vi "CONFIG FILE MAIN Unitest.vi"(0 "File Path":path, 1 "WRITE /READ SECTION":string, 2 "READ KEY":string, 3 "WRITE KEY":string, 4 "WRITE VALUE":string, 5 "error in":errorcluster, 6 "file name":string=".ini", 7 "PARAMETER/CONFIG":bool, 8 "Config Enum":T1) -> (15 "READ VALUE":string, 19 "error out":errorcluster)   [LabVIEW 2025]
uses:
  Config file  FGV Unitest enum.ctl
  <vilib>/Utility/config.llb/Read Key (String).vi
  <vilib>/Utility/config.llb/Write Key (String).vi
  <vilib>/Utility/config.llb/NI_LVConfig.lvlib
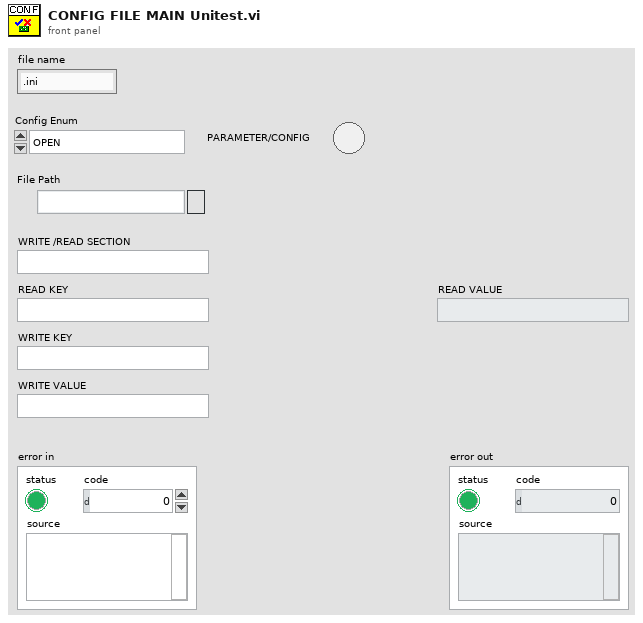
[diagram p1: front panel]
types:
  T1 = typedef "Config file  FGV Unitest enum.ctl" = enum16{"OPEN", "READ", "WRITE", "CLOSE"}
  T2 = typedef "NI_LVConfig.lvlib/Config Data RefNum.ctl" = refnum<k1>
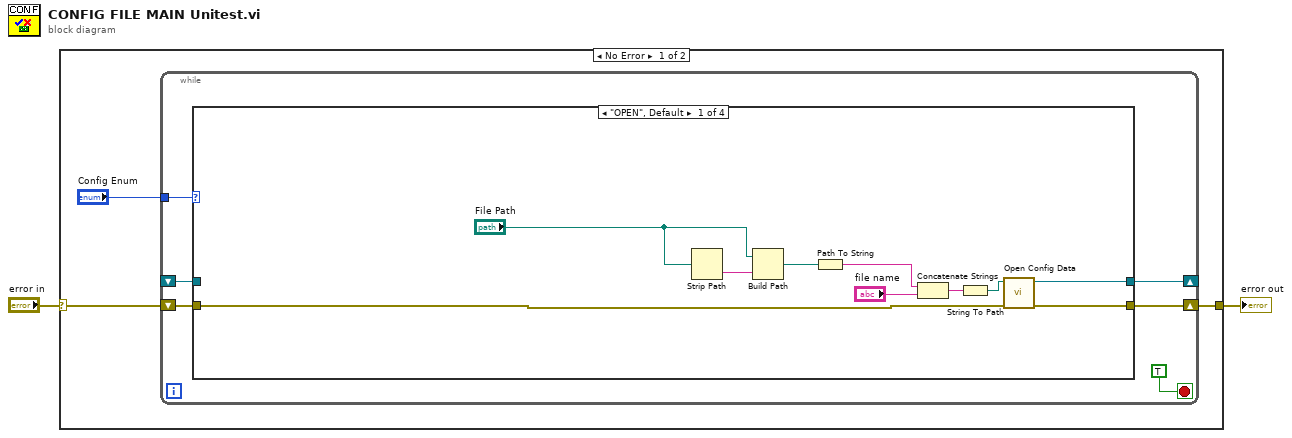
[diagram p0: block diagram]
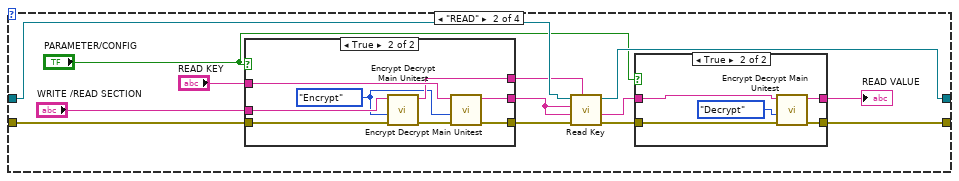
[diagram p2: hidden frame]
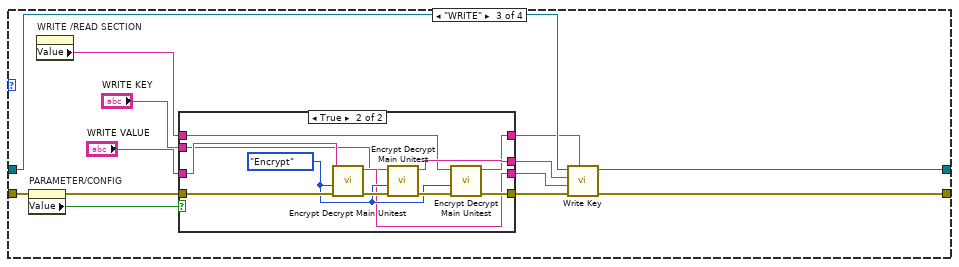
[diagram p5: hidden frame]
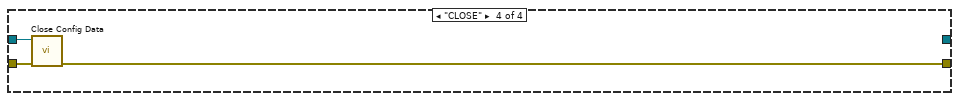
[diagram p7: hidden frame]
diagram:
  n1 = case shown="No Error" "error in" {
    selector: "error in" -> [w4 _]
    tunnel: [w3 _] -> w1
    frame No Error {
      n2 = while {
        tunnel: "Config Enum" -> [w11]
        shift-right: [w9] -> w3
        shift-left: w4 -> [w10]
        shift-right: [w8] -> _
        shift-left: _ -> [w6]
        stop <- TRUE stop-if-true
        n3 = case shown="\"OPEN\", Default" w11 {
          tunnel: w10 -> [w21 w32 w55 w83]
          tunnel: [w20 w25 w64 w81] -> w9
          tunnel: [w19 w33 w63 _] -> w8
          tunnel: w6 -> [_ w34 w65 w82]
          frame "OPEN", Default {
            n4 = Strip Path(path="File Path") -> (name=w13:string)  [unwired: 1 out]
            n5 = Build Path(base path="File Path", name or relative path=w13) -> (appended path=w12:path)
            n6 = Path To String(path=w12) -> (string=w18:string)
            n7 = Concatenate Strings(w18, "file name") -> (w16:string)
            n8 = String To Path(string=w16) -> (path=w15:path)
            n9 = call <vilib>:"Open Config Data.vi"("error in (no error)"=w21, "configuration file path"=w15) -> ("error out"=w20:errorcluster, "refnum"=w19:T2)  [unwired: 7 in, 1 out]
          }
          frame "READ" {
            n10 = case shown="True" "PARAMETER/CONFIG" {
              tunnel: w32 -> [w35 w45]
              tunnel: [w35 w43] -> w31
              tunnel: [w36 w42] -> w30
              tunnel: "READ KEY" -> [w36 w41]
              tunnel: [w37 w40] -> w28
              tunnel: "WRITE /READ SECTION" -> [w37 w39]
              frame False {
              }
              frame True {
                w38 = enum16{"Decrypt", "Encrypt"}."Encrypt" ("Process")
                n11 = call "Encrypt Decrypt Main Unitest.vi"("error in (no error)"=w45, "Process"=w38, "Input"=w39) -> ("error out"=w44:errorcluster, "Output"=w40:string)  [unwired: 7 in]
                n12 = call "Encrypt Decrypt Main Unitest.vi"("error in (no error)"=w44, "Process"=w38, "Input"=w41) -> ("error out"=w43:errorcluster, "Output"=w42:string)  [unwired: 7 in]
              }
            }
            n13 = call-poly <vilib>:"Read Key.vi"("section"=w28, "error in (no error)"=w31, "default value"=w30, "key"=w30, "refnum"=w34) -> ("error out"=w26:errorcluster, "value"=w24:string, "refnum out"=w33:T2)  [unwired: 3 in, 1 out]
            n14 = case shown="True" "PARAMETER/CONFIG" {
              tunnel: w26 -> [w47 w52]
              tunnel: [w47 w51] -> w25
              tunnel: w24 -> [w46 w50]
              tunnel: [w46 w49] -> w23
              frame False {
              }
              frame True {
                n15 = call "Encrypt Decrypt Main Unitest.vi"("error in (no error)"=w52, "Process"=enum16{"Decrypt", "Encrypt"}."Decrypt", "Input"=w50) -> ("error out"=w51:errorcluster, "Output"=w49:string)  [unwired: 7 in]
              }
            }
            "READ VALUE" <- w23
          }
          frame "WRITE" {
            n16 = property on="PARAMETER/CONFIG" class="Bool (strict)"(error in=w55) -> (error out=w54:errorcluster, "Value"=w53:bool)  [unwired: 1 in, 1 out]
            n17 = property on="WRITE /READ SECTION" class="Str"() -> ("Value"=w57:string)  [unwired: 2 in, 2 out]
            n18 = case shown="True" w53 {
              tunnel: w54 -> [w66 w80]
              tunnel: [w66 w77] -> w62
              tunnel: [w67 w75] -> w61
              tunnel: "WRITE VALUE" -> [w67 w74]
              tunnel: [w68 w73] -> w59
              tunnel: "WRITE KEY" -> [w68 w72]
              tunnel: w57 -> [w69 w71]
              tunnel: [w69 w70] -> w56
              frame False {
              }
              frame True {
                w76 = enum16{"Decrypt", "Encrypt"}."Encrypt" ("Process")
                n19 = call "Encrypt Decrypt Main Unitest.vi"("error in (no error)"=w80, "Process"=w76, "Input"=w74) -> ("error out"=w79:errorcluster, "Output"=w75:string)  [unwired: 7 in]
                n20 = call "Encrypt Decrypt Main Unitest.vi"("error in (no error)"=w79, "Process"=w76, "Input"=w72) -> ("error out"=w78:errorcluster, "Output"=w73:string)  [unwired: 7 in]
                n21 = call "Encrypt Decrypt Main Unitest.vi"("error in (no error)"=w78, "Process"=w76, "Input"=w71) -> ("error out"=w77:errorcluster, "Output"=w70:string)  [unwired: 7 in]
              }
            }
            n22 = call-poly <vilib>:"Write Key.vi"("section"=w56, "error in (no error)"=w62, "value"=w61, "key"=w59, "refnum"=w65) -> ("error out"=w64:errorcluster, "refnum out"=w63:T2)  [unwired: 4 in, 1 out]
          }
          frame "CLOSE" {
            n23 = call <vilib>:"Close Config Data.vi"("error in (no error)"=w83, "refnum"=w82) -> ("error out"=w81:errorcluster)  [unwired: 8 in, 1 out]
          }
        }
      }
    }
    frame Error {
    }
  }
  "error out" <- w1
